vi "startVESC.vi"(1 "Baud Rate":T1(ring), 2 "MXP Port":enum16{"A", "B"}(ring)) -> (0 "SPI Config Out":T2)   [LabVIEW 2019]
uses:
  SPI/SPI Config.ctl
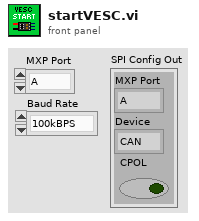
[diagram p1: front panel]
types:
  T1 = enum16{"100kBPS", "250kBPS", "500kBPS", "1000kBPS"}
  T2 = typedef "SPI Config.ctl" = cluster{"MXP Port":enum16{"A", "B"}, "Device":enum16{"CAN", "ENC", "IMU1", "IMU2"}, "CPOL":bool}
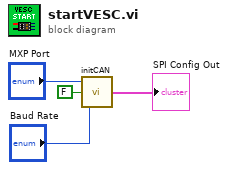
[diagram p0: block diagram]
diagram:
  n1 = call "initCAN.vi"("Baud Rate"="Baud Rate", "CPOL"=FALSE, "MXP Port"="MXP Port") -> ("SPI Config Out"=→"SPI Config Out":T2)
